vi "Execute Locate in Project.vi"(6 "Mouse Position":T1 caption="鼠标位置", 8 "User VI Ref":refnum<vi> caption="用户VI引用", 9 "Menu Item Tag Suffix":string caption="菜单项标签后缀", 10 "Remaining Items":refnum<vi>[](array[refnum]) caption="剩余项", 11 "Affected Items":T2 caption="受影响的项") -> (0 "Fail transaction?":bool caption="操作失败？")   [LabVIEW 2020]
doc: "该VI属于修改LabVIEW快捷菜单部分。这是用户选择快捷菜单时调用的执行VI。该VI执行选中菜单项的操作。"
uses:
  Locate in Project.ctl
  <vilib>/Utility/miscctls.llb/LVPositionTypeDef.ctl
panel:
  # "除“受影响的项”之外，前面板上的其他所有控件都已锁定，以防被意外编辑。修改控件名称或类型，而不是“受影响的项”簇的元素将使VI无法作为菜单插件使用。\n\n请参考每个控件的即时帮助了解其用法。"
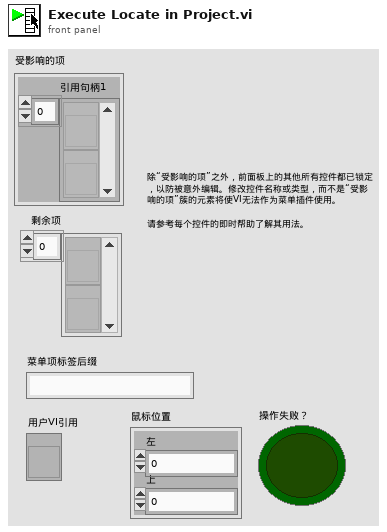
[diagram p1: front panel]
types:
  T1 = typedef "LVPositionTypeDef.ctl" = cluster{"Left":i32, "Top":i32}
  T2 = typedef "Locate in Project.ctl" = cluster{"Refnums 1":refnum<vi>[]}
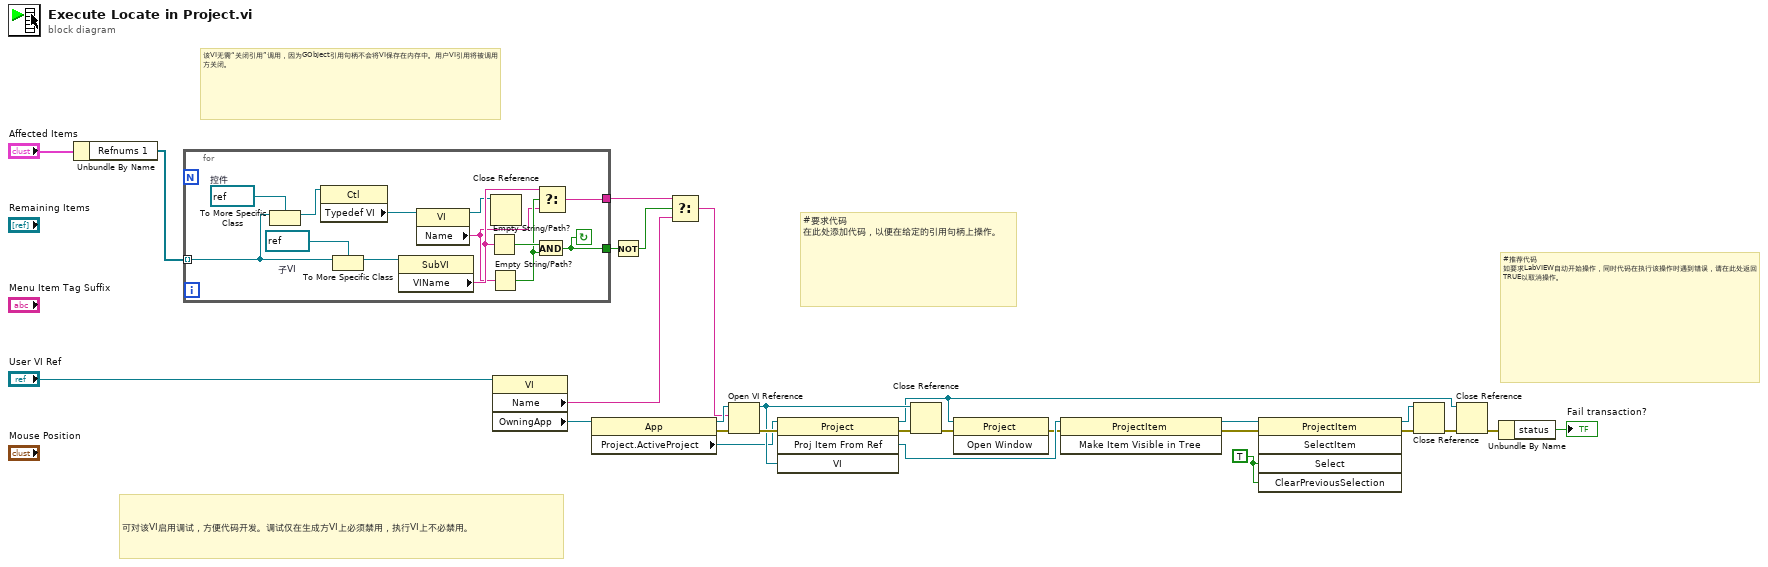
[diagram p0: block diagram]
diagram:
  w13 = TRUE ("Select")
  # "可对该VI启用调试，方便代码开发。调试仅在生成方VI上必须禁用，执行VI上不必禁用。"
  # "#推荐代码 如要求LabVIEW自动开始操作，同时代码在执行该操作时遇到错误，请在此处返回TRUE以取消操作。"
  # "#要求代码 在此处添加代码，以便在给定的引用句柄上操作。"
  # "该VI无需“关闭引用”调用，因为GObject引用句柄不会将VI保存在内存中。用户VI引用将被调用方关闭。"
  n1 = Unbundle By Name("Affected Items") -> ("Refnums 1"=w26:refnum<vi>[])
  n2 = for {
    tunnel: w26 -> [w38] mode=indexing
    tunnel: [w30] -> w6
    tunnel: [w29] -> w4
    stop <- w30 continue-if-true
    w39 = refnum<vi> refnum  # 控件
    w40 = refnum<vi> refnum  # 子VI
    n3 = To More Specific Class(target class=w39, reference=w38) -> (specific class reference=w37:refnum<vi>)  [unwired: 1 in, 1 out]
    n4 = property class="Ctl"(reference=w37) -> ("Typedef VI"=w35:refnum<vi>)  [unwired: 1 in, 2 out]
    n5 = To More Specific Class(target class=w40, reference=w38) -> (specific class reference=w36:refnum<vi>)  [unwired: 1 in, 1 out]
    n6 = property class="SubVI"(reference=w36) -> ("VIName"=w32:string)  [unwired: 1 in, 2 out]
    n7 = property class="VI"(reference=w35) -> (reference out=w28:refnum<vi>, "Name"=w31:string)  [unwired: 1 in, 1 out]
    n8 = Empty String/Path?(string/path=w32) -> (empty?=w34:bool)
    n9 = Empty String/Path?(string/path=w31) -> (empty?=w33:bool)
    n10 = Close Reference(reference=w28) -> ()  [unwired: 1 in, 1 out]
    n11 = And(x=w34, y=w33) -> (x .and. y?=w30:bool)
    n12 = Select(t=w32, s=w33, f=w31) -> (s? t:f=w29:string)
  }
  n13 = property class="VI"(reference="User VI Ref") -> ("Name"=w2:string, "OwningApp"=w24:refnum<vi>)  [unwired: 1 in, 2 out]
  n14 = property class="App"(reference=w24) -> (reference out=w15:refnum<vi>, error out=w1:errorcluster, "Project.ActiveProject"=w16:refnum<vi>)  [unwired: 1 in]
  n15 = Not(x=w6) -> (.not. x?=w5:bool)
  n16 = Select(t=w4, s=w5, f=w2) -> (s? t:f=w3:string)
  n17 = Open VI Reference(application reference (local)=w15, vi path=w3, error in (no error)=w1) -> (vi reference=w20:refnum<vi>, error out=w23:errorcluster)  [unwired: 3 in]
  n18 = invoke class="Project" method="Proj Item From Ref"(reference=w16, error in=w23, "VI"=w20) -> (reference out=w18:refnum<vi>, error out=w22:errorcluster, "ProjItemFromRef"=w19:refnum<vi>)  [unwired: 1 in, 1 out]
  n19 = Close Reference(reference=w20, error in (no error)=w22) -> (error out=w21:errorcluster)
  n20 = invoke class="Project" method="Open Window"(reference=w18, error in=w21) -> (error out=w11:errorcluster)  [unwired: 1 in, 2 out]
  n21 = invoke class="ProjectItem" method="Make Item Visible in Tree"(reference=w19, error in=w11) -> (reference out=w14:refnum<vi>, error out=w12:errorcluster)  [unwired: 1 in, 1 out]
  n22 = invoke class="ProjectItem" method="SelectItem"(reference=w14, error in=w12, "Select"=w13, "ClearPreviousSelection"=w13) -> (reference out=w10:refnum<vi>, error out=w9:errorcluster)  [unwired: 1 in, 3 out]
  n23 = Close Reference(reference=w10, error in (no error)=w9) -> (error out=w17:errorcluster)
  n24 = Close Reference(reference=w18, error in (no error)=w17) -> (error out=w8:errorcluster)
  n25 = Unbundle By Name(w8) -> ("status"=→"Fail transaction?":bool)
